vi "BuildApplication.vi"(4 "Path to project":path) -> (0 "error out":errorcluster, 1 "Generated files":path[](array[path]))   [LabVIEW 2018]
uses:
  <vilib>/AppBuilder/AB_API_Simple/Build (path).vi
  <vilib>/AppBuilder/AB_API_Simple/NI_App_Builder_API.lvlib
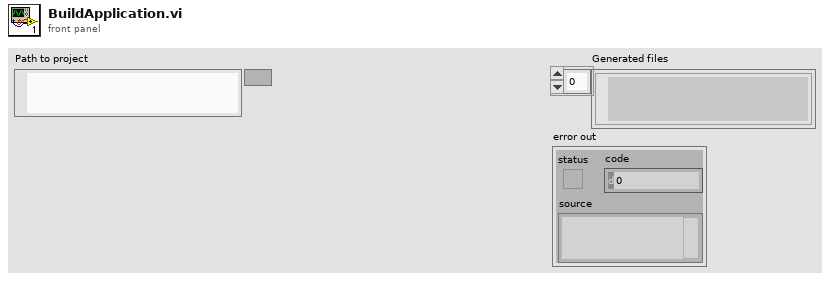
[diagram p1: front panel]
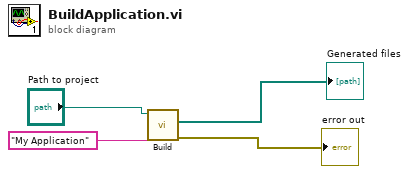
[diagram p0: block diagram]
diagram:
  n1 = call-poly <vilib>:"Build.vi"("Name of build specification (if empty: build all)"="My Application", "Path to project"="Path to project") -> ("error out"=→"error out":errorcluster, "Generated files"=→"Generated files":path[])  [unwired: 8 in]
